vi "oax_Load Data.vi"(0 "File Path (.dat)":path, 1 "Enum":T1(ring)=enum."Load tachless file", 5 "Tacho File Path (.wav)":path, 7 "Simulated speed Path (.ssp)":path, 9 "Vibration File Path (.wav)":path, 11 "error in":errorcluster, 12 "tacho info":T3 {"slope (Rising)" items=["Rising", "Falling"]}) -> (4 "Vibration signals":waveform(dbl)[](array[waveform]), 6 "speed profile":T2 {"speed [RPM]" format="%.2f"; "time [s]" format="%.2f"}, 10 "pulse / rev":i32, 14 "Fs":dbl, 15 "error out":errorcluster)   [LabVIEW 2017]
doc: "Specify the .dat file to load vibration and tachometer data from."
uses:
  <vilib>/addons/Sound and Vibration/Order Analysis/Tach Process/SubVIs/speed profile.ctl
  <vilib>/addons/Sound and Vibration/svt_Calibration/SVL Scale Voltage to EU (N Ch - N Info).vi
  <vilib>/addons/Sound and Vibration/svt_Calibration/SVL Scale Voltage to EU (1 Ch).vi
  <vilib>/addons/_NISVFA/_Shared subVIs/Common/svc_Set SV Channel Info.vi
  <vilib>/addons/_NISVFA/_Shared subVIs/Common/svc_Set SV Channel Info (variant).vi
  <vilib>/addons/_NISVFA/_Shared subVIs/Common/SVL Set dB Reference (variant).vi
  <vilib>/sound2/lvsound2.llb/Sound File Read (DBL).vi
  <vilib>/sound2/lvsound2.llb/Sound File Read Open.vi
  <vilib>/addons/Sound and Vibration/Order Analysis/Tach Process/OAT Analog Tacho Process (1 Tacho).vi
  <vilib>/addons/_NISVFA/_Shared subVIs/Common/svc_Caller VI Returned in Error Source.vi
  <vilib>/addons/_NISVFA/_Shared subVIs/Common/svc_Engineering Units to Unit Label.vi
  <vilib>/addons/_NISVFA/_Shared subVIs/Common/svc_Set dB ref if Pascal.vi
  <vilib>/addons/_NISVFA/_Shared subVIs/Common/svc_Compute Scale Factor to Convert C to EU.vi
  <vilib>/addons/_NISVFA/_Shared subVIs/Common/svc_Compute Scale Factor to Convert V to EU.vi
  <vilib>/addons/Sound and Vibration/Order Analysis/Tach Process/SoundVib_TachProcess.lvlib
  <vilib>/addons/Sound and Vibration/svt_Calibration/SoundVib_Calibration.lvlib
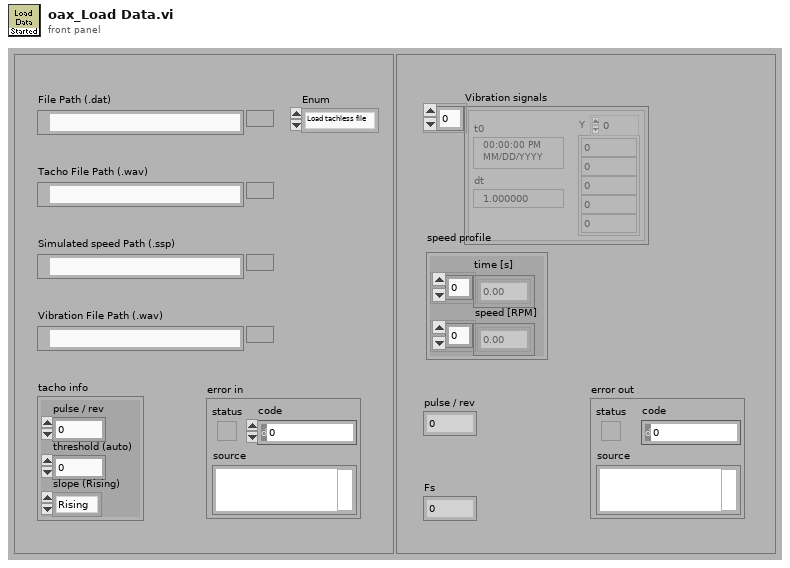
[diagram p1: front panel]
types:
  T1 = enum16{"Load .wav file", "Load .dat file", "Load tachless file", "Load .ssp file"}
  T2 = typedef "SoundVib_TachProcess.lvlib/speed profile.ctl" = cluster{"time [s]":dbl[], "speed [RPM]":dbl[]}
  T3 = cluster{"pulse / rev":i32, "threshold (auto)":dbl, "slope (Rising)":u16}
  T4 = typedef "Sound File Refnum.ctl" = refnum<file>
  T5 = typedef "svc_Channel Info.ctl" = cluster{"sensor sensitivity":dbl, "engineering units":T6, "dB reference":dbl, "custom label":string, "weighting filter":T7, "pregain":dbl}
  T6 = typedef "svc_Engineering Units Text Ring.ctl" = u16
  T7 = typedef "svc_Weighting Filter Text Ring.ctl" = u16
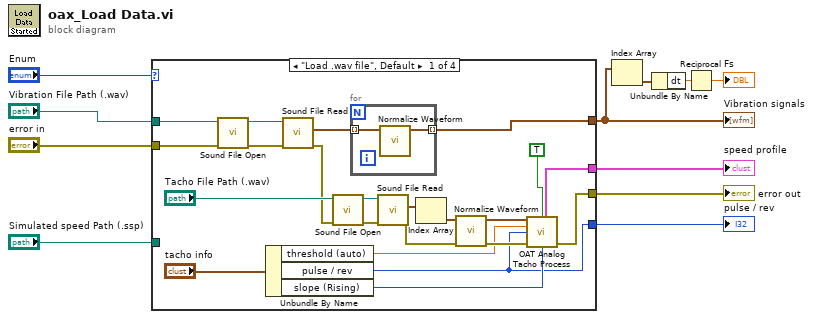
[diagram p0: block diagram]
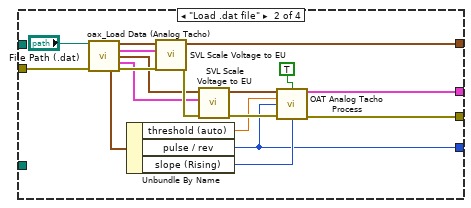
[diagram p2: hidden frame]
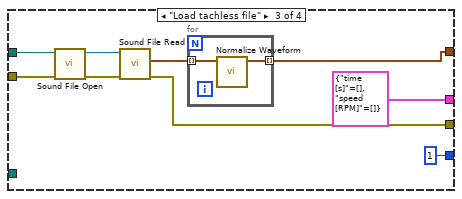
[diagram p3: hidden frame]
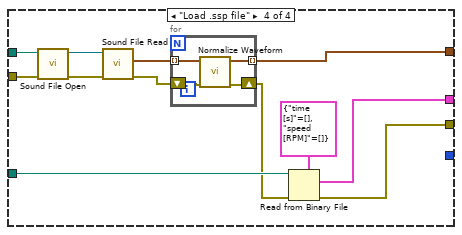
[diagram p4: hidden frame]
diagram:
  n1 = case shown="\"Load .wav file\", Default" "Enum" {
    tunnel: [w13 w45 w58 w71] -> w5
    tunnel: [w23 w44 T2 {"time [s]"=[], "speed [RPM]"=[]} ("speed profile") w67] -> w9
    tunnel: [w16 w43 w56 w65] -> w11
    tunnel: "error in" -> [w28 w41 w57 w72]
    tunnel: [w14 w37 1 ("pulse / rev") _] -> w8
    tunnel: "Vibration File Path (.wav)" -> [w12 _ w59 w73]
    tunnel: "Simulated speed Path (.ssp)" -> [_ _ _ w69]
    frame "Load .wav file", Default {
      n2 = call-poly <vilib>:"Sound File Open.vi"("error in (no error)"=w28, "path"=w12) -> ("error out"=w33:errorcluster, "sound file refnum"=w32:T4)  [unwired: 8 in]
      n3 = Unbundle By Name("tacho info") -> ("threshold (auto)"=w18:dbl, "pulse / rev"=w14:i32, "slope (Rising)"=w24:u16)
      n4 = call-poly <vilib>:"Sound File Read.vi"("error in (no error)"=w33, "sound file refnum"=w32) -> ("error out"=w27:errorcluster, "data"=w17:waveform(dbl)[])  [unwired: 5 in, 3 out]
      n5 = call-poly <vilib>:"Sound File Open.vi"("error in (no error)"=w27, "path"="Tacho File Path (.wav)") -> ("error out"=w31:errorcluster, "sound file refnum"=w29:T4)  [unwired: 8 in]
      n6 = for {
        tunnel: w17 -> [w35] mode=indexing
        tunnel: [w34] -> w13 mode=indexing
        n7 = call <vilib>:"Normalize Waveform.vi"("waveform in"=w35) -> ("normalized waveform"=w34:waveform(dbl))  [unwired: 7 in, 3 out]
      }
      n8 = call-poly <vilib>:"Sound File Read.vi"("error in (no error)"=w31, "sound file refnum"=w29) -> ("error out"=w19:errorcluster, "data"=w25:waveform(dbl)[])  [unwired: 5 in, 3 out]
      n9 = Index Array(array=w25) -> (element=w22:waveform(dbl))  [unwired: 1 in]
      n10 = call <vilib>:"Normalize Waveform.vi"("error in (no error)"=w19, "waveform in"=w22) -> ("error out"=w20:errorcluster, "normalized waveform"=w21:waveform(dbl))  [unwired: 6 in, 2 out]
      n11 = call-poly <vilib>:"OAT Analog Tacho Process.vi"("analog tacho signal"=w21, "reset? (F)"=TRUE, "threshold (auto)"=w18, "pulse/revolution (1)"=w14, "error in (no error)"=w20, "slope (Rising)"=w24) -> ("speed profile"=w23:T2, "error out"=w16:errorcluster)  [unwired: 5 in, 3 out]
    }
    frame "Load .dat file" {
      n12 = call <vilib>:"oax_Load Data (Analog Tacho).vi"("Data Path In"="File Path (.dat)", "error in (no error)"=w41) -> ("vibration data"=w50:waveform(dbl)[], "vibration channel info"=w49:T5[], "analog tacho signal"=w48:waveform(dbl), "tacho channel info"=w47:T5, "tacho info"=w40:T3, "error out"=w52:errorcluster)  [unwired: 7 in, 1 out]
      n13 = Unbundle By Name(w40) -> ("threshold (auto)"=w39:dbl, "pulse / rev"=w37:i32, "slope (Rising)"=w38:u16)
      n14 = call-poly <vilib>:"SVL Scale Voltage to EU.vi"("error in (no error)"=w52, "channel info"=w49, "signals [V]"=w50) -> ("error out"=w53:errorcluster, "scaled signals [EU]"=w45:waveform(dbl)[])  [unwired: 6 in, 1 out]
      n15 = call-poly <vilib>:"SVL Scale Voltage to EU.vi"("error in (no error)"=w53, "channel info"=w47, "signal [V]"=w48) -> ("error out"=w51:errorcluster, "scaled signal [EU]"=w46:waveform(dbl))  [unwired: 6 in, 1 out]
      n16 = call-poly <vilib>:"OAT Analog Tacho Process.vi"("analog tacho signal"=w46, "reset? (F)"=TRUE, "threshold (auto)"=w39, "pulse/revolution (1)"=w37, "error in (no error)"=w51, "slope (Rising)"=w38) -> ("speed profile"=w44:T2, "error out"=w43:errorcluster)  [unwired: 5 in, 3 out]
    }
    frame "Load tachless file" {
      n17 = call-poly <vilib>:"Sound File Open.vi"("error in (no error)"=w57, "path"=w59) -> ("error out"=w62:errorcluster, "sound file refnum"=w61:T4)  [unwired: 8 in]
      n18 = call-poly <vilib>:"Sound File Read.vi"("error in (no error)"=w62, "sound file refnum"=w61) -> ("error out"=w56:errorcluster, "data"=w60:waveform(dbl)[])  [unwired: 5 in, 3 out]
      n19 = for {
        tunnel: w60 -> [w64] mode=indexing
        tunnel: [w63] -> w58 mode=indexing
        n20 = call <vilib>:"Normalize Waveform.vi"("waveform in"=w64) -> ("normalized waveform"=w63:waveform(dbl))  [unwired: 7 in, 3 out]
      }
    }
    frame "Load .ssp file" {
      n21 = call-poly <vilib>:"Sound File Open.vi"("error in (no error)"=w72, "path"=w73) -> ("error out"=w76:errorcluster, "sound file refnum"=w75:T4)  [unwired: 8 in]
      n22 = call-poly <vilib>:"Sound File Read.vi"("error in (no error)"=w76, "sound file refnum"=w75) -> ("error out"=w70:errorcluster, "data"=w74:waveform(dbl)[])  [unwired: 5 in, 3 out]
      n23 = for {
        tunnel: w74 -> [w80] mode=indexing
        tunnel: [w79] -> w71 mode=indexing
        shift-right: [w77] -> w66
        shift-left: w70 -> [w78]
        n24 = call <vilib>:"Normalize Waveform.vi"("error in (no error)"=w78, "waveform in"=w80) -> ("error out"=w77:errorcluster, "normalized waveform"=w79:waveform(dbl))  [unwired: 6 in, 2 out]
      }
      n25 = Read from Binary File(5:T2 {"time [s]"=[], "speed [RPM]"=[]} ("speed profile"), 8:w66, 11:w69) -> (0:w65:errorcluster, 2:w67:T2)  [unwired: 3 in, 2 out]
    }
  }
  "error out" <- w11
  "Vibration signals" <- w5
  "speed profile" <- w9
  "pulse / rev" <- w8
  n26 = Index Array(array=w5) -> (element=w6:waveform(dbl))  [unwired: 1 in]
  n27 = Unbundle By Name(w6) -> ("dt"=w7:dbl)
  n28 = Reciprocal(x=w7) -> (1/x=→"Fs":dbl)
